vi "Convert to Module Class.vi"(8 "error in":errorcluster, 10 "slot ref in":T1 format="%.0x", 11 "SD Module in":refnum<class "SD Module.lvclass">) -> (0 "error out":errorcluster, 2 "module":refnum<class "Module.lvclass">, 3 "SD Module out":refnum<class "SD Module.lvclass">)   [LabVIEW 2017, in "Modules.lvlib" / "SD Module.lvclass"]
uses:
  SD Module.lvclass
  C:/Users/nitest/Documents/niveristand-scan-engine-module-libraries/Source/RSI Module/RSI Module.lvclass
  niveristand-scan-engine-ethercat-custom-device/Custom Device Source/Scripting/Modules/Module/Module.lvclass
  <vilib>/NI Veristand/Custom Device API/Custom Device Item Ref.ctl
  niveristand-scan-engine-ethercat-custom-device/Custom Device Source/Scripting/Modules/Mode Classes/Digital Output Mode/Digital Output Mode.lvclass
  niveristand-scan-engine-ethercat-custom-device/Custom Device Source/Scripting/Modules/Mode Classes/Counter Driven Output Mode/Counter Driven Output Mode.lvclass
  niveristand-scan-engine-ethercat-custom-device/Custom Device Source/Scripting/Modules/Mode Classes/PWM Mode/PWM Mode.lvclass
  RSI Module/RSI Module.lvclass
  <vilib>/NI Veristand/Custom Device Tools/Custom Device Utility Library/Custom Device Utility Library.lvlib
  <vilib>/NI Veristand/Custom Device API/Custom Device API.lvlib
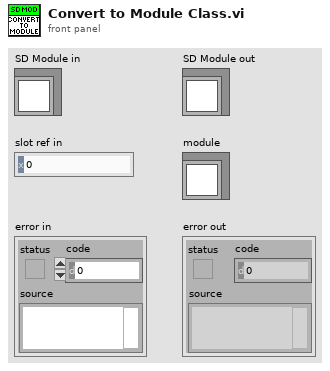
[diagram p1: front panel]
types:
  T1 = typedef "Custom Device API.lvlib/Custom Device Item Ref.ctl" = u64
  T2 = typedef "Custom Device API.lvlib/Custom Device Channel.ctl" = cluster{"Type":T3, "Units":string, "Default Value":dbl, "Faultable":bool, "Scalable":bool}
  T3 = typedef "Custom Device API.lvlib/Custom Device Channel Type.ctl" = enum16{"Input", "Output"}
  T4 = typedef "Modules.lvlib/RSI Module.lvclass/Channels.ctl" = cluster{"# Input Channels":i32, "# Output Channels":i32, "Channel Type":T5, "Units":string}
  T5 = typedef "Modules.lvlib/RSI Module.lvclass/Channel Type.ctl" = enum16{"Analog", "Digital"}
  T6 = typedef "Scan Engine Scripting.lvlib/digital channel settings.ctl" = cluster{"name":string, "default value":bool}
  T7 = typedef "Modules.lvlib/SD Module.lvclass/CDO.ctl" = cluster{"Drive From Slot":u32, "CDO Channels":T8[]}
  T8 = typedef "Modules.lvlib/SD Module.lvclass/CDO Channel.ctl" = cluster{"Counter driven enabled":bool}
  T9 = typedef "Scan Engine Scripting.lvlib/counter driven output channel settings.ctl" = cluster{"name":string, "default value":bool, "counter driven state":T10}
  T10 = typedef "Scan Engine Scripting.lvlib/Counter Driven Output Channel.lvclass/Counter Driven State.ctl" = enum16{"Disabled", "Enabled"}
  T11 = typedef "Modules.lvlib/SD Module.lvclass/PWM.ctl" = cluster{"PWM Channels":T12[]}
  T12 = typedef "Modules.lvlib/SD Module.lvclass/PWM Channel.ctl" = cluster{"PWM frequency":u32}
  T13 = typedef "Scan Engine Scripting.lvlib/pwm channel settings.ctl" = cluster{"name":string, "default value":dbl, "frequency":T14}
  T14 = typedef "Scan Engine Scripting.lvlib/PWM Output Channel.lvclass/Frequency.ctl" = enum16{"1 Hz (1,000,000 us)", "50 Hz (20,000 us)", "250 Hz (4,000 us)", "500 Hz (2,000 us)", "1 kHz (1,000 us)", "5 kHz (200 us)", "10 kHz (100 us)", "20 kHz (50 us)"}
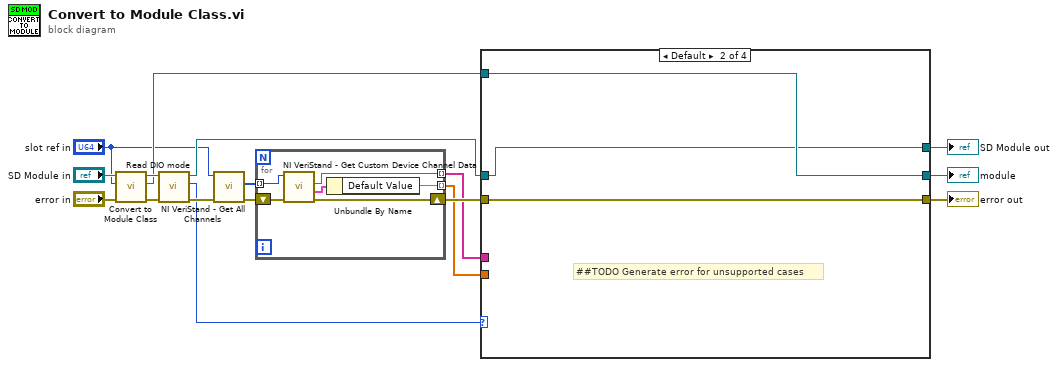
[diagram p0: block diagram]
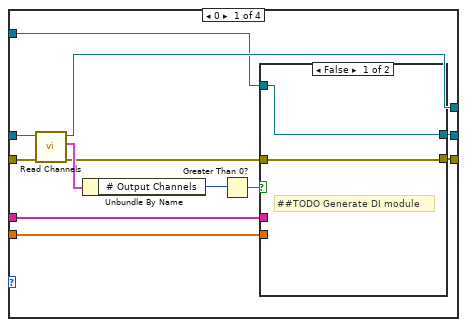
[diagram p2: hidden frame]
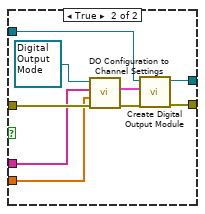
[diagram p3: hidden frame]
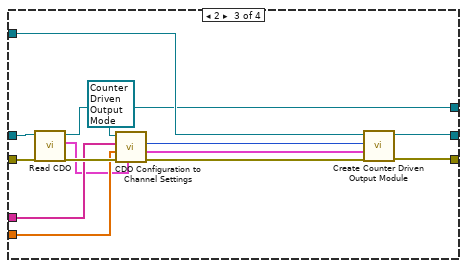
[diagram p4: hidden frame]
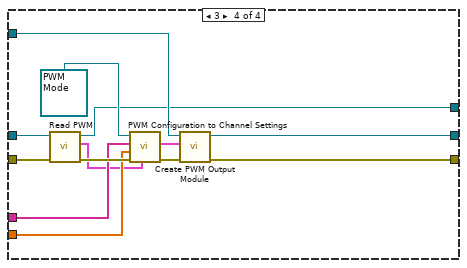
[diagram p5: hidden frame]
diagram:
  n1 = call-parent "Convert to Module Class.vi"("error in"="error in", "slot ref in"="slot ref in", "RSI Module in"="SD Module in") -> ("error out"=w10:errorcluster, "module"=w5:refnum<class "Module.lvclass">, "RSI Module out"=w12:refnum<class "SD Module.lvclass">)  [unwired: 6 in]
  n2 = call "Read DIO mode.vi"("error in (no error)"=w10, "SD Module in"=w12) -> ("error out"=w15:errorcluster, "DIO mode"=w14:u32, "SD Module out"=w8:refnum<class "SD Module.lvclass">)  [unwired: 7 in]
  n3 = call <vilib>:"NI VeriStand - Get All Channels.vi"("error in"=w15, "Section Ref in"="slot ref in") -> ("error out"=w16:errorcluster, "Channel Refs"=w17:T1[])  [unwired: 6 in, 2 out]
  n4 = for {
    tunnel: w17 -> [w22] mode=indexing
    shift-right: [w19] -> w9
    shift-left: w16 -> [w23]
    tunnel: [w21] -> w7 mode=indexing
    tunnel: [w18] -> w6 mode=indexing
    n5 = call <vilib>:"NI VeriStand - Get Custom Device Channel Data.vi"("error in (no error)"=w23, "Channel Ref in"=w22) -> ("error out"=w19:errorcluster, "Channel"=w20:T2, "Channel Name"=w21:string)  [unwired: 4 in, 3 out]
    n6 = Unbundle By Name(w20) -> ("Default Value"=w18:dbl)
  }
  n7 = case shown="Default" w14 {
    tunnel: w9 -> [w35 w49 w63 w74]
    tunnel: w8 -> [w34 w47 w62 w75]
    tunnel: w7 -> [w28 _ w60 w72]
    tunnel: w6 -> [w27 _ w59 w71]
    tunnel: w5 -> [w26 w48 w55 w67]
    tunnel: [w25 w49 w54 w66] -> w2
    tunnel: [w24 w48 w52 w65] -> w4
    tunnel: [w29 w47 w53 w64] -> w3
    frame 0 {
      n8 = call "Read Channels.vi"("error in (no error)"=w35, "RSI Module in"=w34) -> ("error out"=w30:errorcluster, "Channels"=w33:T4, "RSI Module out"=w29:refnum<class "SD Module.lvclass">)  [unwired: 7 in]
      n9 = Unbundle By Name(w33) -> ("# Output Channels"=w32:i32)
      n10 = Greater Than 0?(x=w32) -> (x > 0?=w31:bool)
      n11 = case shown="False" w31 {
        tunnel: w30 -> [w37 w45]
        tunnel: w28 -> [_ w44]
        tunnel: w27 -> [_ w43]
        tunnel: w26 -> [w36 w40]
        tunnel: [w37 w39] -> w25
        tunnel: [w36 w38] -> w24
        frame False {
          # "##TODO Generate DI module"
        }
        frame True {
          n12 = call-dynamic "DO Configuration to Channel Settings.vi"("error in"=w45, "default values"=w43, "names"=w44, "digital output mode in"=refnum<class "Digital Output Mode.lvclass"> refnum ("Scan Engine Scripting.lvlib:Digital Output Mode.lvclass")) -> ("error out"=w42:errorcluster, "channel settings"=w41:T6[])  [unwired: 5 in, 1 out]
          n13 = call-dynamic "Create Digital Output Module.vi"("error in"=w42, "channel settings"=w41, "module in"=w40) -> ("error out"=w39:errorcluster, "module out"=w38:refnum<class "Module.lvclass">)  [unwired: 7 in]
        }
      }
    }
    frame Default {
      # "##TODO Generate error for unsupported cases"
    }
    frame 2 {
      n14 = call-dynamic "Read CDO.vi"("error in (no error)"=w63, "SD Module in"=w62) -> ("error out"=w61:errorcluster, "CDO"=w58:T7, "SD Module out"=w53:refnum<class "SD Module.lvclass">)  [unwired: 7 in]
      n15 = call-dynamic "CDO Configuration to Channel Settings.vi"("CDO"=w58, "error in"=w61, "default values"=w59, "names"=w60, "Counter Driven Output Mode in"=refnum<class "Counter Driven Output Mode.lvclass"> refnum ("Scan Engine Scripting.lvlib:Counter Driven Output Mode.lvclass")) -> ("error out"=w56:errorcluster, "channel settings"=w50:T9[], "drive from slot"=w51:u32)  [unwired: 3 in, 1 out]
      n16 = call-dynamic "Create Counter Driven Output Module.vi"("error in"=w56, "channel settings"=w50, "drive from slot"=w51, "module in"=w55) -> ("error out"=w54:errorcluster, "module out"=w52:refnum<class "Module.lvclass">)  [unwired: 6 in]
    }
    frame 3 {
      n17 = call-dynamic "Read PWM.vi"("error in (no error)"=w74, "SD Module in"=w75) -> ("error out"=w73:errorcluster, "PWM"=w70:T11, "SD Module out"=w64:refnum<class "SD Module.lvclass">)  [unwired: 7 in]
      n18 = call-dynamic "PWM Configuration to Channel Settings.vi"("PWM"=w70, "error in"=w73, "default values"=w71, "names"=w72, "PWM Mode in"=refnum<class "PWM Mode.lvclass"> refnum ("Scan Engine Scripting.lvlib:PWM Mode.lvclass")) -> ("error out"=w69:errorcluster, "channel settings"=w68:T13[])  [unwired: 4 in, 1 out]
      n19 = call "Create PWM Output Module.vi"("error in (no error)"=w69, "channel settings"=w68, "module in"=w67) -> ("error out"=w66:errorcluster, "module out"=w65:refnum<class "Module.lvclass">)  [unwired: 7 in]
    }
  }
  "error out" <- w2
  "SD Module out" <- w3
  "module" <- w4
